vi "ESP32_Socket_NoLoop.vi"() -> ()   [LabVIEW 2022 SP3]
doc: "Demonstrates how to open a connection to an TCP server, read the data being sent, and display the data on a chart. This VI is designed to stop if the TCP connection is terminated."
panel:
  out "data out":string
  in  "address":string="10.0.0.127"
  in  "Server Closed":string="The server VI closed the connection."
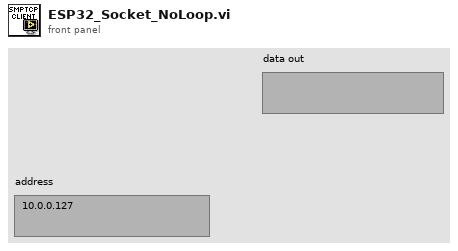
[diagram p1: front panel]
types:
  T1 = enum16{"Standard", "Buffered", "CRLF", "Immediate"}
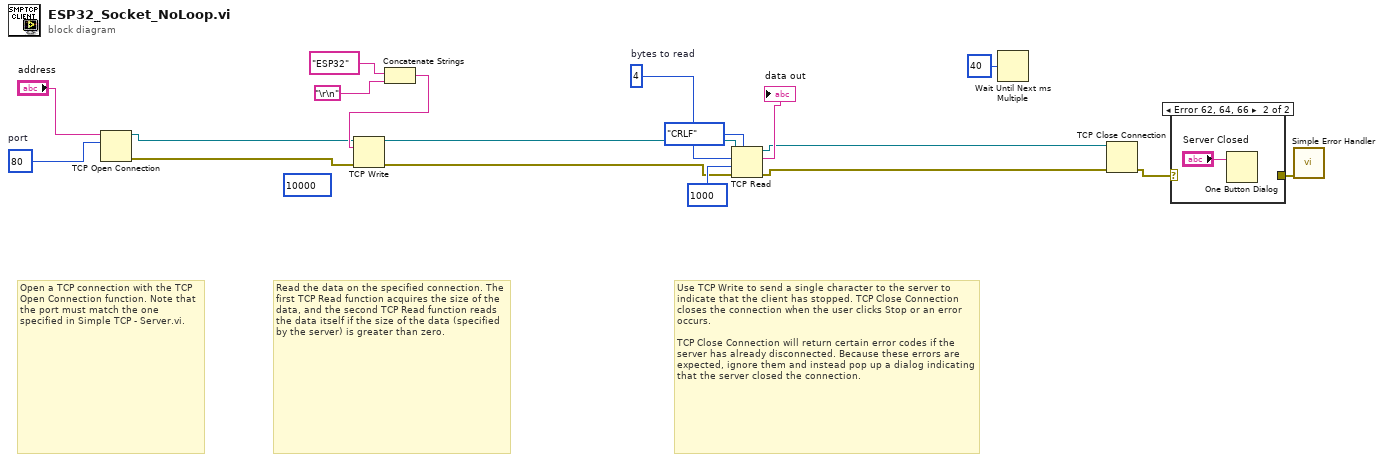
[diagram p0: block diagram]
diagram:
  (unwired) 10000 ("timeout ms (25000)")
  w14 = 4  # bytes to read
  w16 = u16 80  # port
  # "Use TCP Write to send a single character to the server to indicate that the client has stopped. TCP Close Connection closes the connection when the user clicks Stop or an error occurs.\n\nTCP Close Connection will return certain error codes if the server has already disconnected. Because these errors are expected, ignore them and instead pop up a dialog indicating that the server closed the connection."
  # "Read the data on the specified connection. The first TCP Read function acquires the size of the data, and the second TCP Read function reads the data itself if the size of the data (specified by the server) is greater than zero."
  # "Open a TCP connection with the TCP Open Connection function. Note that the port must match the one specified in Simple TCP - Server.vi."
  n1 = TCP Open Connection(address="address", remote port or service name=w16) -> (connection ID=w4:refnum<k5>, error out=w3:errorcluster)  [unwired: 3 in]
  n2 = Concatenate Strings("ESP32" ("data in"), "\r\n") -> (w6:string)
  n3 = TCP Write(connection ID=w4, data in=w6, error in (no error)=w3) -> (connection ID out=w11:refnum<k5>, error out=w5:errorcluster)  [unwired: 1 in, 1 out]
  n4 = TCP Read(connection ID=w11, bytes to read=w14, error in (no error)=w5, 7:T1."CRLF" ("mode (standard)"), 9:1000 ("timeout ms (25000)")) -> (connection ID out=w2:refnum<k5>, data out=→"data out":string, error out=w1:errorcluster)
  n5 = Wait Until Next ms Multiple(millisecond multiple=u32 40) -> ()  [unwired: 1 out]
  n6 = TCP Close Connection(connection ID=w2, error in (no error)=w1) -> (error out=w17:errorcluster)  [unwired: 1 in, 1 out]
  n7 = case shown="Error 62, 64, 66" w17 {
    selector: w17 -> [w19 _]
    tunnel: [w19 _] -> w18
    frame #0 {
    }
    frame #1 {
      n8 = One Button Dialog(message="Server Closed") -> ()  [unwired: 1 in, 1 out]
    }
  }
  n9 = call <vilib>:"Simple Error Handler.vi"("error in (no error)"=w18) -> ()  [unwired: 4 in, 5 out]
